vi "Cleanup References.vi"(8 "Error In":errorcluster, 11 "Appearance Actor in":refnum<class "Appearance Actor.lvclass">) -> (0 "Error Out":errorcluster, 3 "Appearance Actor out":refnum<class "Appearance Actor.lvclass">)   [LabVIEW 2021, in "Appearance Actor.lvlib" / "Appearance Actor.lvclass"]
uses:
  Appearance Actor.lvclass
  Appearance Actor.lvclass/Appearance Actor.ctl
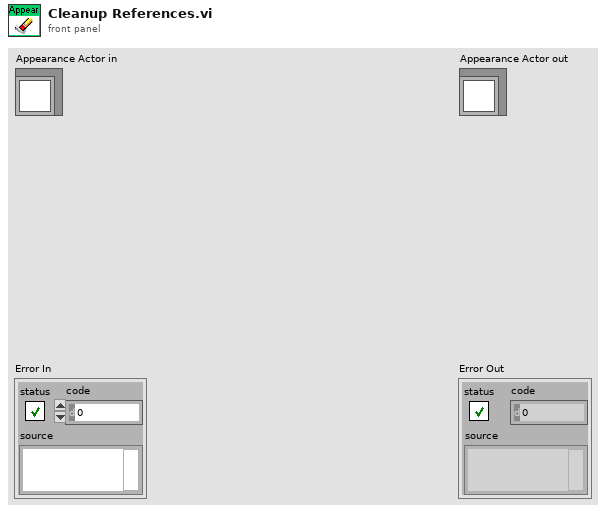
[diagram p1: front panel]
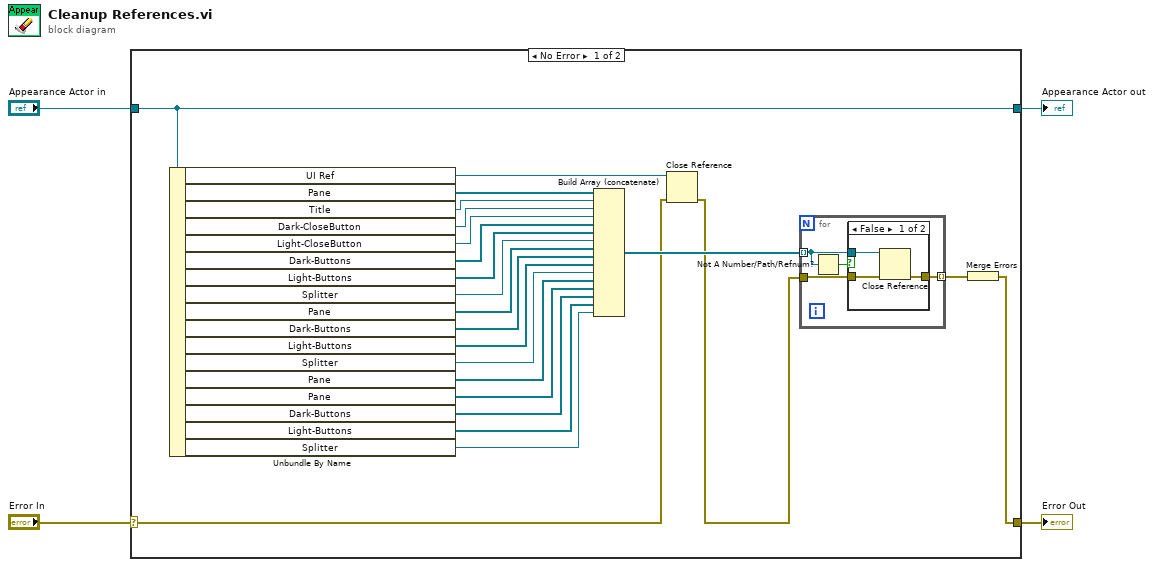
[diagram p0: block diagram]
diagram:
  n1 = case shown="No Error" "Error In" {
    selector: "Error In" -> [w8 w37]
    tunnel: [w5 w37] -> w3
    tunnel: [w27 w36] -> w1
    tunnel: "Appearance Actor in" -> [w27 w36]
    frame No Error {
      n2 = Unbundle By Name(w27) -> ("UI Ref"=w9:refnum<vi>, "Pane"=w26:refnum<vi>[], "Title"=w25:refnum<vi>, "Dark-CloseButton"=w24:refnum<vi>, "Light-CloseButton"=w23:refnum<vi>, "Dark-Buttons"=w22:refnum<vi>[], "Light-Buttons"=w21:refnum<vi>[], "Splitter"=w20:refnum<vi>, "Pane"=w19:refnum<vi>[], "Dark-Buttons"=w18:refnum<vi>[], "Light-Buttons"=w17:refnum<vi>[], "Splitter"=w16:refnum<vi>, "Pane"=w15:refnum<vi>[], "Pane"=w14:refnum<vi>[], "Dark-Buttons"=w13:refnum<vi>[], "Light-Buttons"=w12:refnum<vi>[], "Splitter"=w11:refnum<vi>)
      n3 = Build Array (concatenate)(w26, w25, w24, w23, w22, w21, w20, w19, w18, w17, w16, w15, w14, w13, w12, w11) -> (w10:refnum<vi>[])
      n4 = Close Reference(reference=w9, error in (no error)=w8) -> (error out=w7:errorcluster)
      n5 = for {
        tunnel: [w31] -> w6 mode=indexing
        tunnel: w7 -> [w30]
        tunnel: w10 -> [w28] mode=indexing
        n6 = Not A Number/Path/Refnum?(number/path/refnum=w28) -> (NaN/Path/Refnum?=w29:bool)
        n7 = case shown="False" w29 {
          tunnel: [w34 w35] -> w31
          tunnel: w30 -> [w33 w35]
          tunnel: w28 -> [w32 _]
          frame False {
            n8 = Close Reference(reference=w32, error in (no error)=w33) -> (error out=w34:errorcluster)
          }
          frame True {
          }
        }
      }
      n9 = Merge Errors(w6) -> (w5:errorcluster)
    }
    frame Error {
    }
  }
  "Error Out" <- w3
  "Appearance Actor out" <- w1
